vi "DesenhoPlanta_ver1.vi"() -> ()   [LabVIEW 2013]
uses:
  <vilib>/measure/NI_MABase.lvlib
panel:
  in  "Slide":dbl(slide) scale=0.0..100.0
  out "Tanque\nInferior":dbl(slide) scale=0.0..100.0
  out "Tanque \nSuperior":dbl(slide) scale=0.0..100.0
  in  "Habilita Escrita\nExcel":bool=TRUE caption="Enable"
  in  "ON/OFF":bool
  in  "stop":bool
  in  "amplitude":dbl=1.0 format="%0.2p"
  in  "frequency":dbl=10.0 format="%0.2p"
  in  "sampling info":cluster{"Fs":dbl, "#s":dbl}={"Fs"=1000.0, "#s"=1000.0} {"Fs" format="%.2p"}
  in  "offset":dbl format="%0.2p"
  in  "signal type":T1(ring)
  out "Waveform Chart":waveform(dbl)(graph)
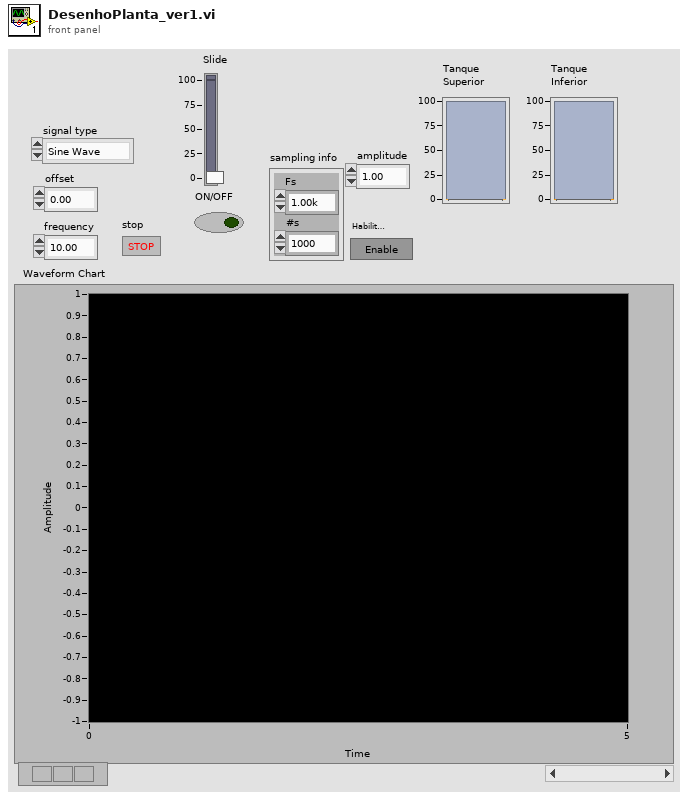
[diagram p1: front panel]
types:
  T1 = enum16{"Sine Wave", "Triangle Wave", "Square Wave", "Sawtooth Wave"}
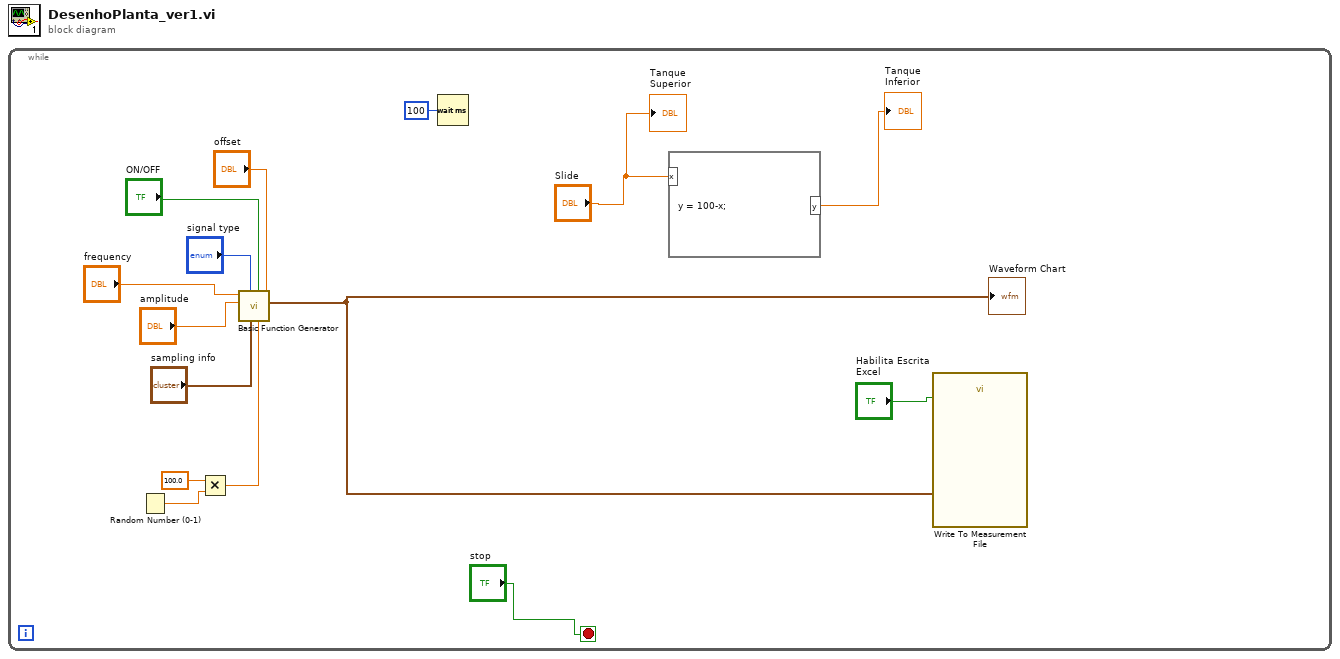
[diagram p0: block diagram]
diagram:
  n1 = while {
    stop <- "stop" stop-if-true
    n2 = Random Number (0-1)() -> (number: 0 to 1=w6:dbl)
    n3 = Multiply(x=100.0, y=w6) -> (x*y=w5:dbl)
    n4 = call <vilib>:"Basic Function Generator.vi"("offset"="offset", "square wave duty cycle (%)"=w5, "reset signal"="ON/OFF", "sampling info"="sampling info", "signal type"="signal type", "amplitude"="amplitude", "frequency"="frequency") -> ("signal out"=w4:waveform(dbl))  [unwired: 2 in, 2 out]
    "Waveform Chart" <- w4
    n5 = Wait (ms)(milliseconds to wait=u32 100) -> ()  [unwired: 1 out]
    n6 = formula code="y = 100-x;"("x"="Slide") -> ("y"=→"Tanque\nInferior":dbl)
    n7 = call "Write To Measurement File"("Signals"=w4, "Enable"="Habilita Escrita\nExcel") -> ()  [unwired: 15 in, 3 out]
    "Tanque \nSuperior" <- "Slide"
  }
